vi "Open Module Refs.vi"(8 "error in (no error)":errorcluster, 11 "RSI Modules in":T1[](array[typedef]) {"Module Config Data"."Config Block Data Refs"."Data Reference" format="%.0x"; "CDOutput Data"."BD Refs"."Data Reference" format="%.0x"; "CDInput Data"."BD Refs"."Data Reference" format="%.0x"; "VS ref" format="%.0x"}) -> (0 "error out":errorcluster, 3 "RSI Modules out":T1[](array[typedef]) {"Module Config Data"."Config Block Data Refs"."Data Reference" format="%.0x"; "CDOutput Data"."BD Refs"."Data Reference" format="%.0x"; "CDInput Data"."BD Refs"."Data Reference" format="%.0x"; "VS ref" format="%.0x"})   [LabVIEW 2016, in "Scan Engine Custom Device.lvlib"]
uses:
  Scan Engine Custom Device.lvlib
  <vilib>/NI Veristand/Custom Device API/Custom Device Item Ref.ctl
  <vilib>/NI Veristand/Custom Device API/Custom Device API.lvlib
  Modules.lvlibp/RSI Module/RSI Module.lvclass
  <vilib>/NI Veristand/Custom Device API/Data Reference.ctl
  <vilib>/NI Veristand/Custom Device API/Block Data Reference.ctl
  Type Defs/Input Data.ctl
  Type Defs/Output Data.ctl
  Type Defs/RSI Module Data.ctl
  Modules.lvlibp/RSI Module/Channel Type.ctl
  Modules.lvlibp/RSI Module/Module Models.ctl
  Type Defs/Module Config Data.ctl
  Type Defs/Mixed IO.ctl
  Type Defs/Open Module IOVs.ctl
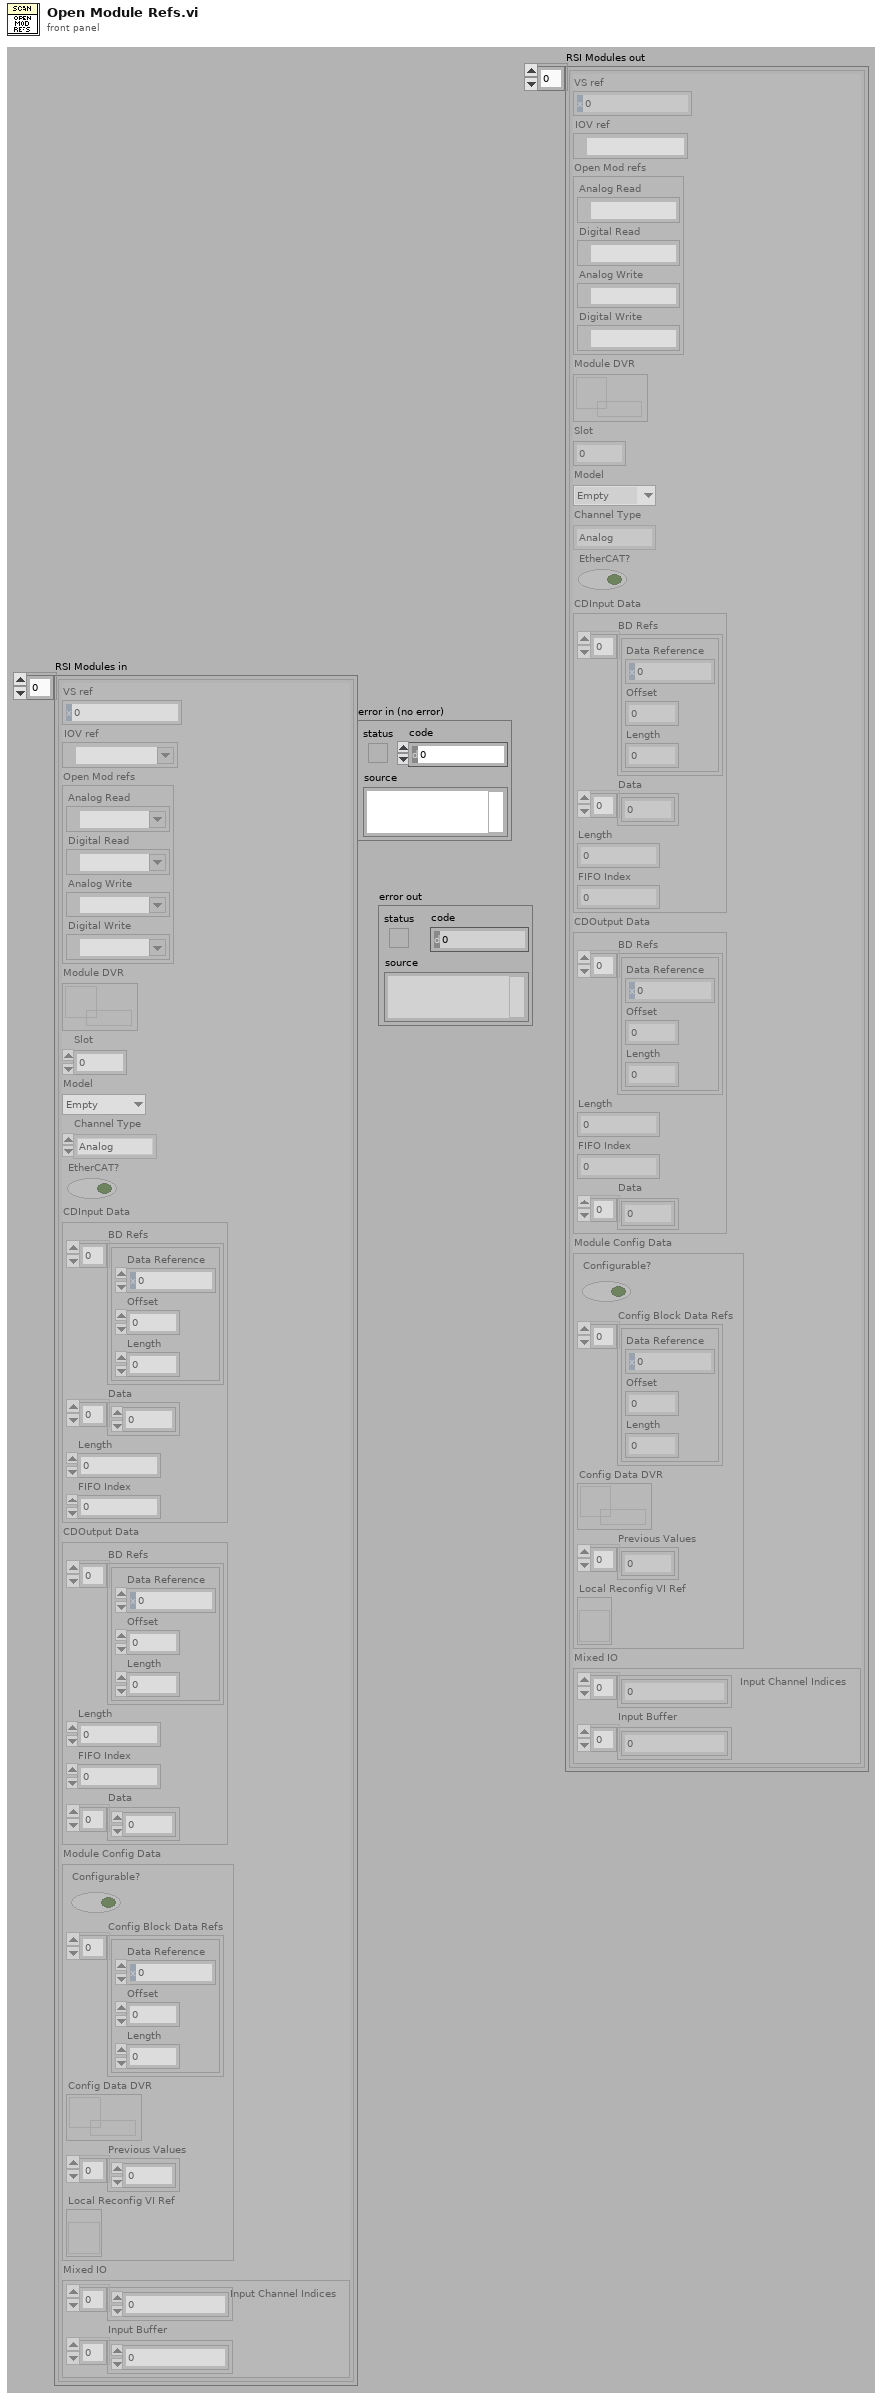
[diagram p1: front panel]
types:
  T1 = typedef "Scan Engine Custom Device.lvlib/RSI Module Data.ctl" = cluster{"VS ref":T2, "IOV ref":refnum<k21>, "Open Mod refs":T3, "Module DVR":refnum<data-value>, "Slot":u32, "Model":T4, "Channel Type":T5, "EtherCAT?":bool, "CDInput Data":T6, "CDOutput Data":T9, "Module Config Data":T10, "Mixed IO":T11}
  T2 = typedef "Custom Device API.lvlib/Custom Device Item Ref.ctl" = u64
  T3 = typedef "Scan Engine Custom Device.lvlib/Open Module IOVs.ctl" = cluster{"Analog Read":refnum<k21>, "Digital Read":refnum<k21>, "Analog Write":refnum<k21>, "Digital Write":refnum<k21>}
  T4 = typedef "Modules.lvlibp/RSI Module.lvclass/Module Models.ctl" = enum16{"Empty", "NI 9201", "NI 9203", "NI 9205", "NI 9206", "NI 9207", "NI 9208", "NI 9211", "NI 9213", "NI 9214", "NI 9215", "NI 9217", "NI 9219", "NI 9221", "NI 9225", "NI 9227", "NI 9229", "NI 9233", "NI 9234", "NI 9235", "NI 9236", "NI 9237", "NI 9239", "NI 9263", "NI 9264", "NI 9265", "NI 9269", "NI 9375", "NI 9401", "NI 9402", "NI 9403", "NI 9411", "NI 9421", "NI 9422", "NI 9423", "NI 9425", "NI 9426", "NI 9435", "NI 9472", "NI 9474", "NI 9475", "NI 9476", "NI 9477", "NI 9478", "NI 9481", "NI 9482", "NI 9485"}
  T5 = typedef "Modules.lvlibp/RSI Module.lvclass/Channel Type.ctl" = enum16{"Analog", "Digital"}
  T6 = typedef "Scan Engine Custom Device.lvlib/Input Data.ctl" = cluster{"BD Refs":T7[], "Data":dbl[], "Length":i32, "FIFO Index":i32}
  T7 = typedef "Custom Device API.lvlib/Block Data Reference.ctl" = cluster{"Data Reference":T8, "Offset":u64, "Length":u64}
  T8 = typedef "Custom Device API.lvlib/Data Reference.ctl" = i32
  T9 = typedef "Scan Engine Custom Device.lvlib/Output Data.ctl" = cluster{"BD Refs":T7[], "Length":i32, "FIFO Index":i32, "Data":dbl[]}
  T10 = typedef "Scan Engine Custom Device.lvlib/Module Config Data.ctl" = cluster{"Configurable?":bool, "Config Block Data Refs":T7[], "Config Data DVR":refnum<data-value>, "Previous Values":dbl[], "Local Reconfig VI Ref":refnum<vi>}
  T11 = typedef "Scan Engine Custom Device.lvlib/Mixed IO.ctl" = cluster{"Input Channel Indices":i32[], "Input Buffer":dbl[]}
  T12 = cluster{"Read Access":enum8{"Allowed", "Required", "None"}, "Write Access":enum8{"Allowed", "Required", "None"}}
  T13 = typedef "Scan Engine Custom Device.lvlib/Module IO Type.ctl" = enum16{"Input", "Output", "Mixed"}
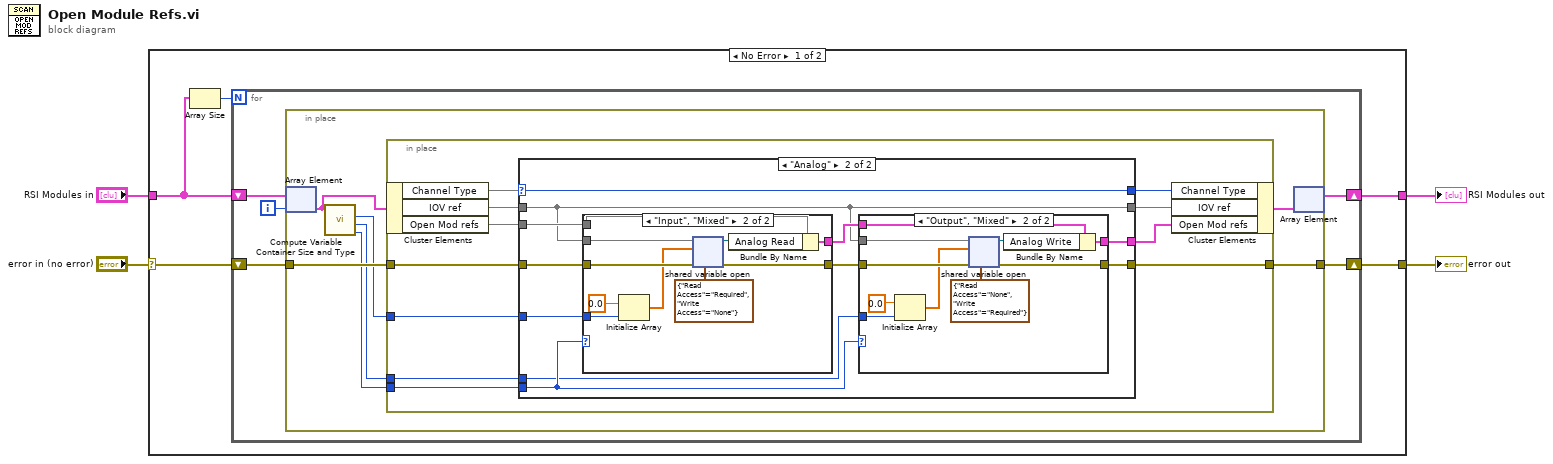
[diagram p0: block diagram]
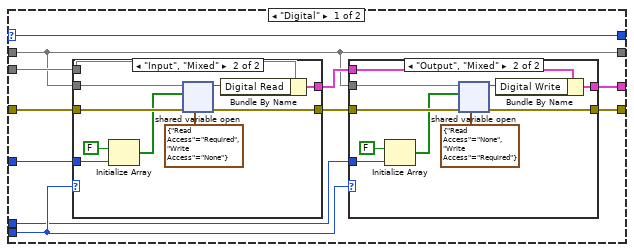
[diagram p2: hidden frame]
diagram:
  n1 = case shown="No Error" "error in (no error)" {
    selector: "error in (no error)" -> [w5 w104]
    tunnel: "RSI Modules in" -> [w8 w103]
    tunnel: [w7 w103] -> w3
    tunnel: [w6 w104] -> w2
    frame No Error {
      n2 = Array Size(array=w8) -> (size(s)=w9:i32)
      n3 = for {
        N: w9 -> [_]
        shift-right: [w10] -> w6
        shift-left: w5 -> [w12]
        shift-right: [w11] -> w7
        shift-left: w8 -> [w14]
        i -> [w13]
        n4 = in-place {
          in-place-border: w12 -> [w21]
          in-place-border: [w20] -> w10
          n5 = in-place-array #1(w14, w13) -> (w15:T1)
          n6 = call "Compute Variable Container Size and Type.vi"("RSI Module in"=w15) -> ("ModIOType"=w18:T13, "Write Session IOV Size"=w17:i32, "Read Session IOV Size"=w16:i32)  [unwired: 8 in]
          n7 = in-place {
            in-place-border: w21 -> [w32]
            in-place-border: [w28] -> w20
            in-place-border: w18 -> [w24]
            in-place-border: w17 -> [w23]
            in-place-border: w16 -> [w22]
            n8 = in-place-cluster #2(w15) -> ("Channel Type"=w26, "IOV ref"=w29, "Open Mod refs"=w31)
            n9 = case shown="\"Analog\"" w26 {
              selector: w26 -> [w41 w76]
              tunnel: w32 -> [w43 w78]
              tunnel: w31 -> [w42 w77]
              tunnel: [w37 w72] -> w30
              tunnel: w29 -> [w37 w72]
              tunnel: [w33 w68] -> w28
              tunnel: [w34 w69] -> w27
              tunnel: [w41 w76] -> w25
              tunnel: w24 -> [w36 w71]
              tunnel: w23 -> [w35 w70]
              tunnel: w22 -> [w40 w75]
              frame "Digital" {
                n10 = case shown="\"Input\", \"Mixed\"" w36 {
                  tunnel: w43 -> [w57 w67]
                  tunnel: [w57 w66] -> w39
                  tunnel: [w56 w65] -> w38
                  tunnel: w42 -> [w56 w64]
                  tunnel: w37 -> [_ w63]
                  tunnel: w40 -> [_ w61]
                  frame "Output" {
                  }
                  frame "Input", "Mixed" {
                    n11 = Initialize Array(FALSE, w61) -> (w59:bool[])
                    n12 = shared-variable-open(w63, w67, w59, T12 {"Read Access"=enum."Required", "Write Access"=enum."None"} ("access")) -> (w62:refnum<k21>, w66:errorcluster)
                    n13 = Bundle By Name(cluster=w64, "Digital Read"=w62) -> (w65:cluster{})
                  }
                }
                n14 = case shown="\"Output\", \"Mixed\"" w36 {
                  tunnel: w39 -> [w44 w55]
                  tunnel: [w44 w54] -> w33
                  tunnel: [w45 w53] -> w34
                  tunnel: w38 -> [w45 w52]
                  tunnel: w37 -> [_ w51]
                  tunnel: w35 -> [_ w49]
                  frame "Input" {
                  }
                  frame "Output", "Mixed" {
                    n15 = Initialize Array(FALSE, w49) -> (w47:bool[])
                    n16 = shared-variable-open(w51, w55, w47, T12 {"Read Access"=enum."None", "Write Access"=enum."Required"} ("access")) -> (w50:refnum<k21>, w54:errorcluster)
                    n17 = Bundle By Name(cluster=w52, "Digital Write"=w50) -> (w53:cluster{})
                  }
                }
              }
              frame "Analog" {
                n18 = case shown="\"Input\", \"Mixed\"" w71 {
                  tunnel: w78 -> [w92 w102]
                  tunnel: [w92 w101] -> w74
                  tunnel: [w91 w100] -> w73
                  tunnel: w77 -> [w91 w99]
                  tunnel: w72 -> [_ w98]
                  tunnel: w75 -> [_ w96]
                  frame "Output" {
                  }
                  frame "Input", "Mixed" {
                    n19 = Initialize Array(0.0, w96) -> (w95:dbl[])
                    n20 = shared-variable-open(w98, w102, w95, T12 {"Read Access"=enum."Required", "Write Access"=enum."None"} ("access")) -> (w97:refnum<k21>, w101:errorcluster)
                    n21 = Bundle By Name(cluster=w99, "Analog Read"=w97) -> (w100:cluster{})
                  }
                }
                n22 = case shown="\"Output\", \"Mixed\"" w71 {
                  tunnel: w74 -> [w79 w90]
                  tunnel: [w79 w89] -> w68
                  tunnel: [w80 w88] -> w69
                  tunnel: w73 -> [w80 w87]
                  tunnel: w72 -> [_ w86]
                  tunnel: w70 -> [_ w84]
                  frame "Input" {
                  }
                  frame "Output", "Mixed" {
                    n23 = Initialize Array(0.0, w84) -> (w83:dbl[])
                    n24 = shared-variable-open(w86, w90, w83, T12 {"Read Access"=enum."None", "Write Access"=enum."Required"} ("access")) -> (w85:refnum<k21>, w89:errorcluster)
                    n25 = Bundle By Name(cluster=w87, "Analog Write"=w85) -> (w88:cluster{})
                  }
                }
              }
            }
            n26 = in-place-cluster #2("Channel Type"=w25, "IOV ref"=w30, "Open Mod refs"=w27) -> (w19:cluster{})
          }
          n27 = in-place-array #1(w19) -> (w11:T1[])  [unwired: 1 out]
        }
      }
    }
    frame Error {
    }
  }
  "RSI Modules out" <- w3
  "error out" <- w2
